vi "simulator_commands.vi"() -> ()   [LabVIEW 2018]
uses:
  mono_commands.ctl
panel:
  out "JSON string":string
  out "data":string
  out "value 3":T1
  out "length 2":u32
  out "value 2":cluster{"magic_number":u32, "length":u32}
  in  "length":u32
  in  "magic_number":u32
  out "data out":string
  out "value":T1
  in  "Simulator Configuration":path=path "C:/Users/celit/Documents/GitHub/client/configurations/simulator.json"
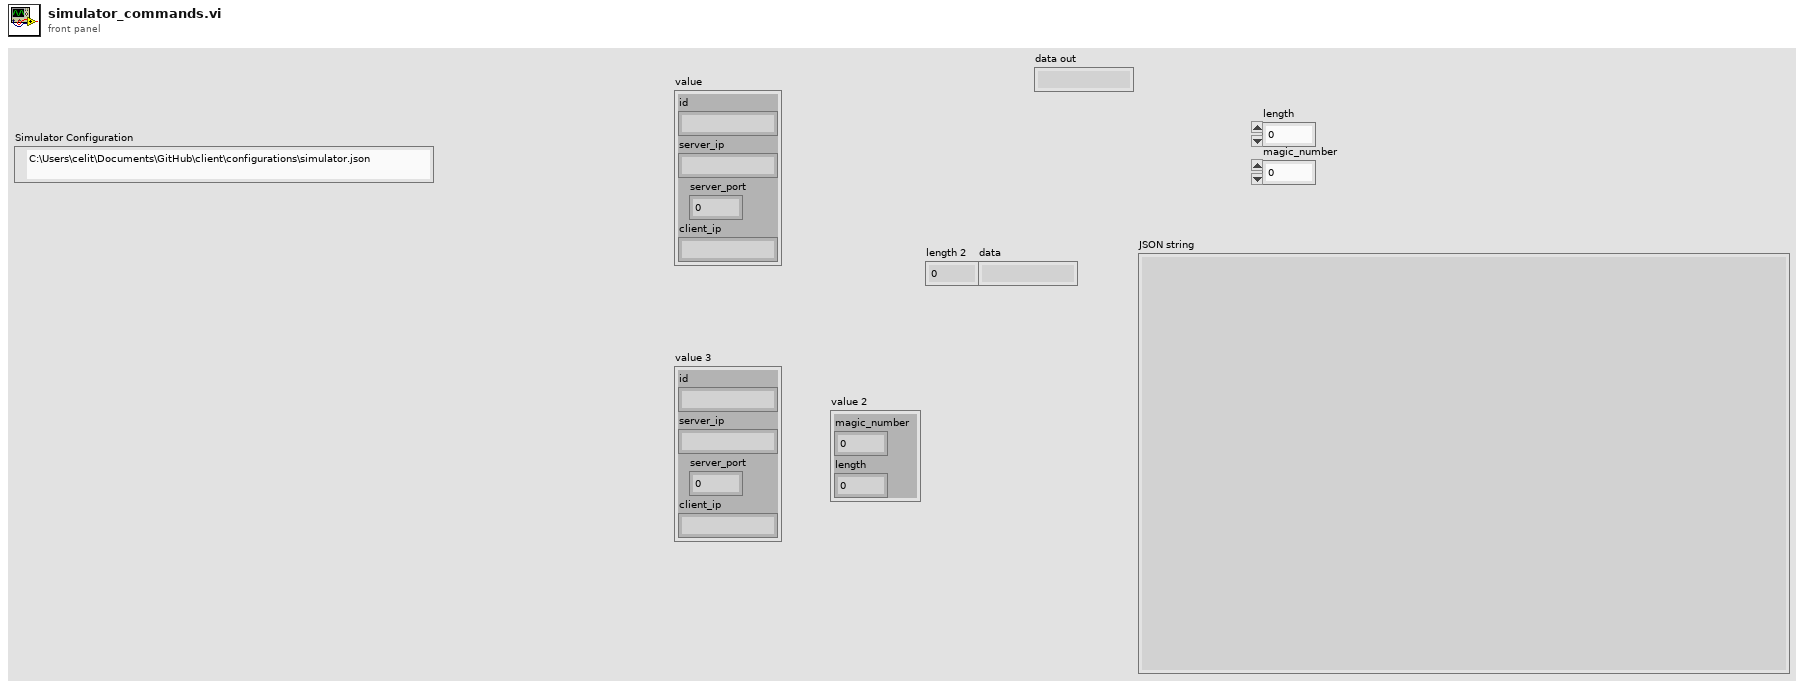
[diagram p1: front panel]
types:
  T1 = cluster{"id":string, "server_ip":string, "server_port":i32, "client_ip":string}
  T2 = cluster{"class":string, "status":i32, "messages":string}
  T3 = typedef "mono_commands.ctl" = cluster{"SIMULATOR_STATUS_UUID":string, "STREAM_DATA_COMMAND_UUID":string, "SIMULATOR_CONFIG_COMMAND_UUID":string, "VEHICLE_CONFIG_COMMAND_UUID":string, "EGO_CONTROL_COMMAND_UID":string, "WAYPOINT_UPDATE_COMMAND_UID":string, "SCENARIO_COMMAND_UID":string, "MAP_COMMAND_UID":string, "SPAWN_COMMAND_UID":string, "MOVE_ACTOR_COMMAND_UID":string, "SCENARIO_INIT_COMMAND_UID":string, "ATTACH_SENSOR_COMMAND_UID":string, "DETACH_SENSOR_COMMAND_UID":string, "CONTROL_HEADER":string, "RESPONSE_HEADER":string}
  T4 = cluster{cluster{"class":string, "status":i32, "messages":string}, string}
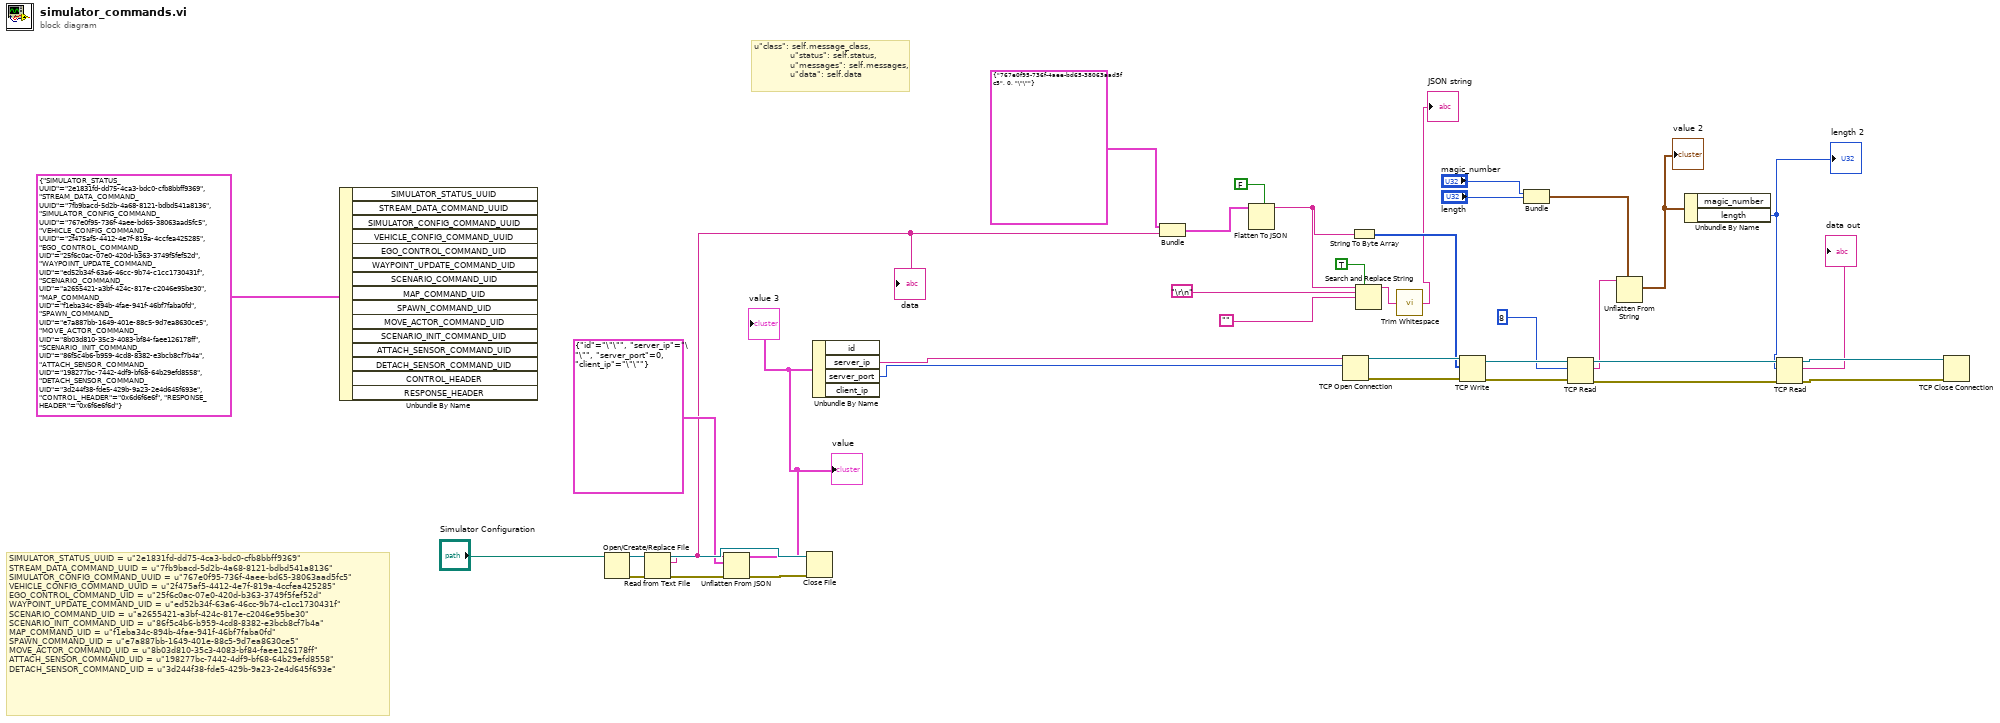
[diagram p0: block diagram]
diagram:
  # "u\"class\": self.message_class,\n            u\"status\": self.status,\n            u\"messages\": self.messages,\n            u\"data\": self.data"
  # "SIMULATOR_STATUS_UUID = u\"2e1831fd-dd75-4ca3-bdc0-cfb8bbff9369\"\nSTREAM_DATA_COMMAND_UUID = u\"7fb9bacd-5d2b-4a68-8121-bdbd541a8136\"\nSIMULATOR_CONFIG_COMMAND_UUID = u\"767e0f95-736f-4aee-bd65-38063aad5fc5\"\nVEHICLE_CONFIG_COMMAND_UUID = u\"2f475af5-4412-4e7f-819a-4ccfea425285\"\nEGO_CONTROL_COMMAND_UID = u\"25f6c0ac-07e0-420d-b363-3749f5fef52d\"\nWAYPOINT_UPDATE_COMMAND_UID = u\"ed52b34f-63a6-46cc-9b74-c1cc1730431f\"\nSCENARIO_COMMAND_UID = u\"a2655421-a3bf-424c-817e-c2046e95be30\"\nSCENARIO_INIT_COMMAND_UID = u\"86f5c4b6-b959-4cd8-8382-e3bcb8cf7b4a\"\nMAP_COMMAND_UID = u\"f1eba34c-894b-4fae-941f-46bf7faba0fd\"\nSPAWN_COMMAND_UID = u\"e7a887bb-1649-401e-88c5-9d7ea8630ce5\"\nMOVE_ACTOR_COMMAND_UID = u\"8b03d810-35c3-4083-bf84-faee126178ff\"\nATTACH_SENSOR_COMMAND_UID = u\"198277bc-7442-4df9-bf68-64b29efd8558\"\nDETACH_SENSOR_COMMAND_UID = u\"3d244f38-fde5-429b-9a23-2e4d645f693e\""
  n1 = Unbundle By Name(T3 {"SIMULATOR_STATUS_UUID"="2e1831fd-dd75-4ca3-bdc0-cfb8bbff9369", "STREAM_DATA_COMMAND_UUID"="7fb9bacd-5d2b-4a68-8121-bdbd541a8136", "SIMULATOR_CONFIG_COMMAND_UUID"="767e0f95-736f-4aee-bd65-38063aad5fc5", "VEHICLE_CONFIG_COMMAND_UUID"="2f475af5-4412-4e7f-819a-4ccfea425285", "EGO_CONTROL_COMMAND_UID"="25f6c0ac-07e0-420d-b363-3749f5fef52d", "WAYPOINT_UPDATE_COMMAND_UID"="ed52b34f-63a6-46cc-9b74-c1cc1730431f", "SCENARIO_COMMAND_UID"="a2655421-a3bf-424c-817e-c2046e95be30", "MAP_COMMAND_UID"="f1eba34c-894b-4fae-941f-46bf7faba0fd", "SPAWN_COMMAND_UID"="e7a887bb-1649-401e-88c5-9d7ea8630ce5", "MOVE_ACTOR_COMMAND_UID"="8b03d810-35c3-4083-bf84-faee126178ff", "SCENARIO_INIT_COMMAND_UID"="86f5c4b6-b959-4cd8-8382-e3bcb8cf7b4a", "ATTACH_SENSOR_COMMAND_UID"="198277bc-7442-4df9-bf68-64b29efd8558", "DETACH_SENSOR_COMMAND_UID"="3d244f38-fde5-429b-9a23-2e4d645f693e", "CONTROL_HEADER"="0x6d6f6e6f", "RESPONSE_HEADER"="0x6f6e6f6d"}) -> ()  [unwired: 15 out]
  n2 = Open/Create/Replace File(file path (use dialog)="Simulator Configuration") -> (refnum out=w38:refnum<file>, error out=w37:errorcluster)  [unwired: 5 in, 1 out]
  n3 = Read from Text File(file (use dialog)=w38, error in=w37) -> (refnum out=w34:refnum<file>, text=w10:string, error out=w35:errorcluster)  [unwired: 2 in, 1 out]
  "data" <- w10
  n4 = Unflatten From JSON(JSON string=w10, type and defaults=T1 {"id"="\"\"", "server_ip"="\"\"", "server_port"=0, "client_ip"="\"\""}, error in (no error)=w35) -> (value=w12:T1, error out=w36:errorcluster)  [unwired: 4 in]
  "value" <- w12
  "value 3" <- w12
  n5 = Close File(refnum=w34, error in=w36) -> ()  [unwired: 2 out]
  n6 = Unbundle By Name(w12) -> ("server_ip"=w29:string, "server_port"=w28:i32)  [unwired: 2 out]
  n7 = Bundle(T2 {"class"="767e0f95-736f-4aee-bd65-38063aad5fc5", "status"=0, "messages"="\"\""}, w10) -> (w7:T4)  [unwired: 1 in]
  n8 = Flatten To JSON(enable LabVIEW extensions? (T)=FALSE, anything=w7) -> (JSON string=w6:string)  [unwired: 1 in, 1 out]
  n9 = TCP Open Connection(address=w29, remote port or service name=w28) -> (connection ID=w31:refnum<k5>, error out=w30:errorcluster)  [unwired: 3 in]
  n10 = String To Byte Array(string=w6) -> (unsigned byte array=w9:u8[])
  n11 = Search and Replace String(replace all?=TRUE ("replace all? (F)"), input string=w6, search string="\r\n", replace string="") -> (result string=w3:string)  [unwired: 4 in, 3 out]
  n12 = call <vilib>:"Trim Whitespace.vi"("string"=w3) -> ("trimmed string"=→"JSON string":string)  [unwired: 1 in]
  n13 = TCP Write(connection ID=w31, data in=w9, error in (no error)=w30) -> (connection ID out=w23:refnum<k5>, error out=w22:errorcluster)  [unwired: 1 in, 1 out]
  n14 = Bundle("magic_number"="magic_number", "length"="length") -> (w15:cluster{"magic_number":u32, "length":u32})  [unwired: 1 in]
  n15 = TCP Read(connection ID=w23, bytes to read=8, error in (no error)=w22) -> (connection ID out=w21:refnum<k5>, data out=w16:string, error out=w20:errorcluster)  [unwired: 2 in]
  n16 = Unflatten From String(type=w15, binary string=w16) -> (value=w14:cluster{"magic_number":u32, "length":u32})  [unwired: 3 in, 2 out]
  "value 2" <- w14
  n17 = Unbundle By Name(w14) -> ("length"=w13:u32)  [unwired: 1 out]
  "length 2" <- w13
  n18 = TCP Read(connection ID=w21, bytes to read=w13, error in (no error)=w20) -> (connection ID out=w27:refnum<k5>, data out=→"data out":string, error out=w26:errorcluster)  [unwired: 2 in]
  n19 = TCP Close Connection(connection ID=w27, error in (no error)=w26) -> ()  [unwired: 1 in, 2 out]
